vi "HandleDb.vi"(8 "error in (no error)":errorcluster, 11 "AnalogComparator in":refnum<class "AnalogComparator.lvclass">) -> (0 "error out":errorcluster, 3 "AnalogComparator out":refnum<class "AnalogComparator.lvclass">)   [LabVIEW 2019, in "AnalogComparator.lvclass"]
uses:
  AnalogComparator.lvclass
  AnalogComparator.lvclass/AnalogComparator.ctl
  Logger_class/EventCode.ctl
  Logger_class/Priority.ctl
  Logger_class/Logger.lvclass
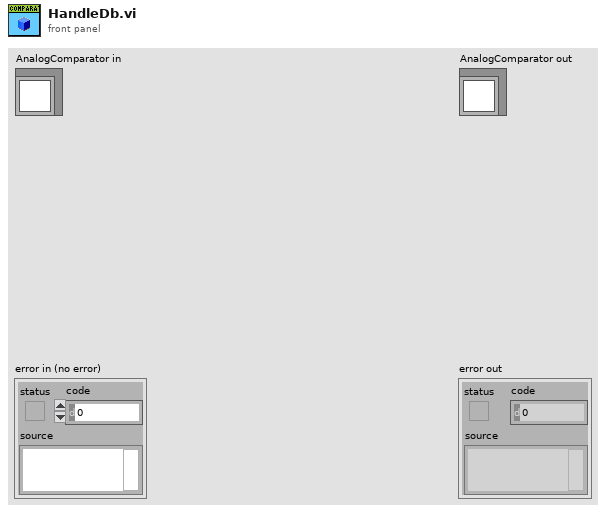
[diagram p1: front panel]
types:
  T1 = typedef "Logger.lvclass/Priority.ctl" = enum16{"Alert", "Critical", "Error", "Warning", "Notice", "Informational", "Debug"}
  T2 = typedef "Logger.lvclass/EventCode.ctl" = enum16{"DI_EU_LO", "DI_EU_HI", "DIO_LO", "DIO_HI", "DI_RAW_LO", "DI_RAW_HI", "DO_LO", "DO_HI", "DA_OK", "DA_ALARM", "AA_HI", "AA_HIHI", "AA_LO", "AA_LOLO", "AA_OK", "CMD", "OUT_OF_RANGE_OK", "OUT_OF_RANGE_LO", "OUT_OF_RANGE_HI", "CONFIG", "DI_LO", "DI_HI"}
  T3 = typedef "Logger.lvclass/EventData.ctl" = cluster{"obj_tag":string, "event_tag":string, "code":T2, "Priority":T1, "Value":dbl, "Description":string, "Time Stamp":timestamp}
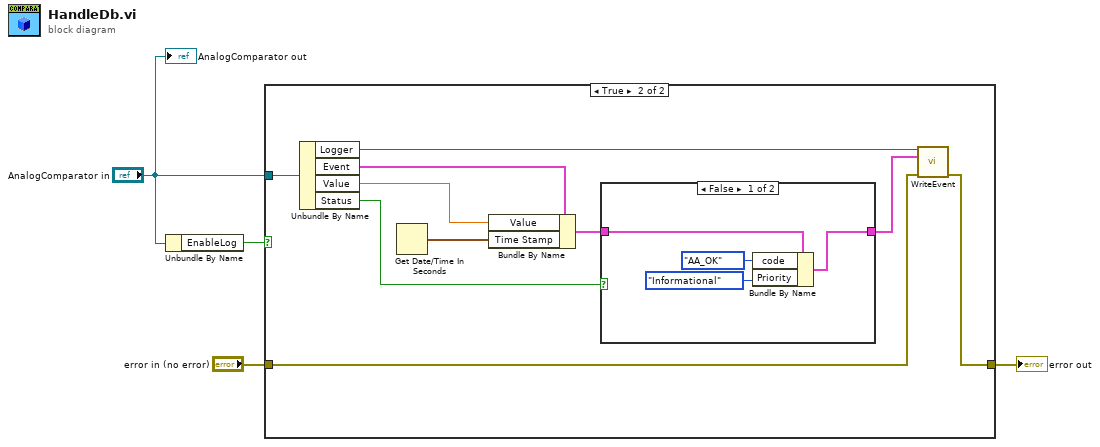
[diagram p0: block diagram]
diagram:
  n1 = Unbundle By Name("AnalogComparator in") -> ("EnableLog"=w1:bool)
  n2 = case shown="True" w1 {
    tunnel: "error in (no error)" -> [w5 w15]
    tunnel: [w5 w14] -> w3
    tunnel: "AnalogComparator in" -> [_ w6]
    frame False {
    }
    frame True {
      n3 = Unbundle By Name(w6) -> ("Logger"=w13:refnum<class "Logger.lvclass">, "Event"=w12:T3, "Value"=w10:dbl, "Status"=w9:bool)
      n4 = Get Date/Time In Seconds() -> (seconds since 1Jan1904=w11:timestamp)
      n5 = Bundle By Name(cluster=w12, "Value"=w10, "Time Stamp"=w11) -> (w7:T3)
      n6 = case shown="False" w9 {
        tunnel: [w18 w20] -> w8
        tunnel: w7 -> [w19 w20]
        frame False {
          n7 = Bundle By Name(cluster=w19, "code"=EventCode."AA_OK", "Priority"=Priority."Informational") -> (w18:T3)
        }
        frame True {
        }
      }
      n8 = call "WriteEvent.vi"("reference in"=w13, "Event"=w8, "error in (no error)"=w15) -> ("error out"=w14:errorcluster)  [unwired: 11 in, 1 out]
    }
  }
  "error out" <- w3
  "AnalogComparator out" <- "AnalogComparator in"
